vi "File read sim.vi"() -> ()   [LabVIEW 2017]
panel:
  out "Angle Array":dbl[](array[numeric])
  out "Distance Array":u32[](array[numeric])
  out "Telegram String":string
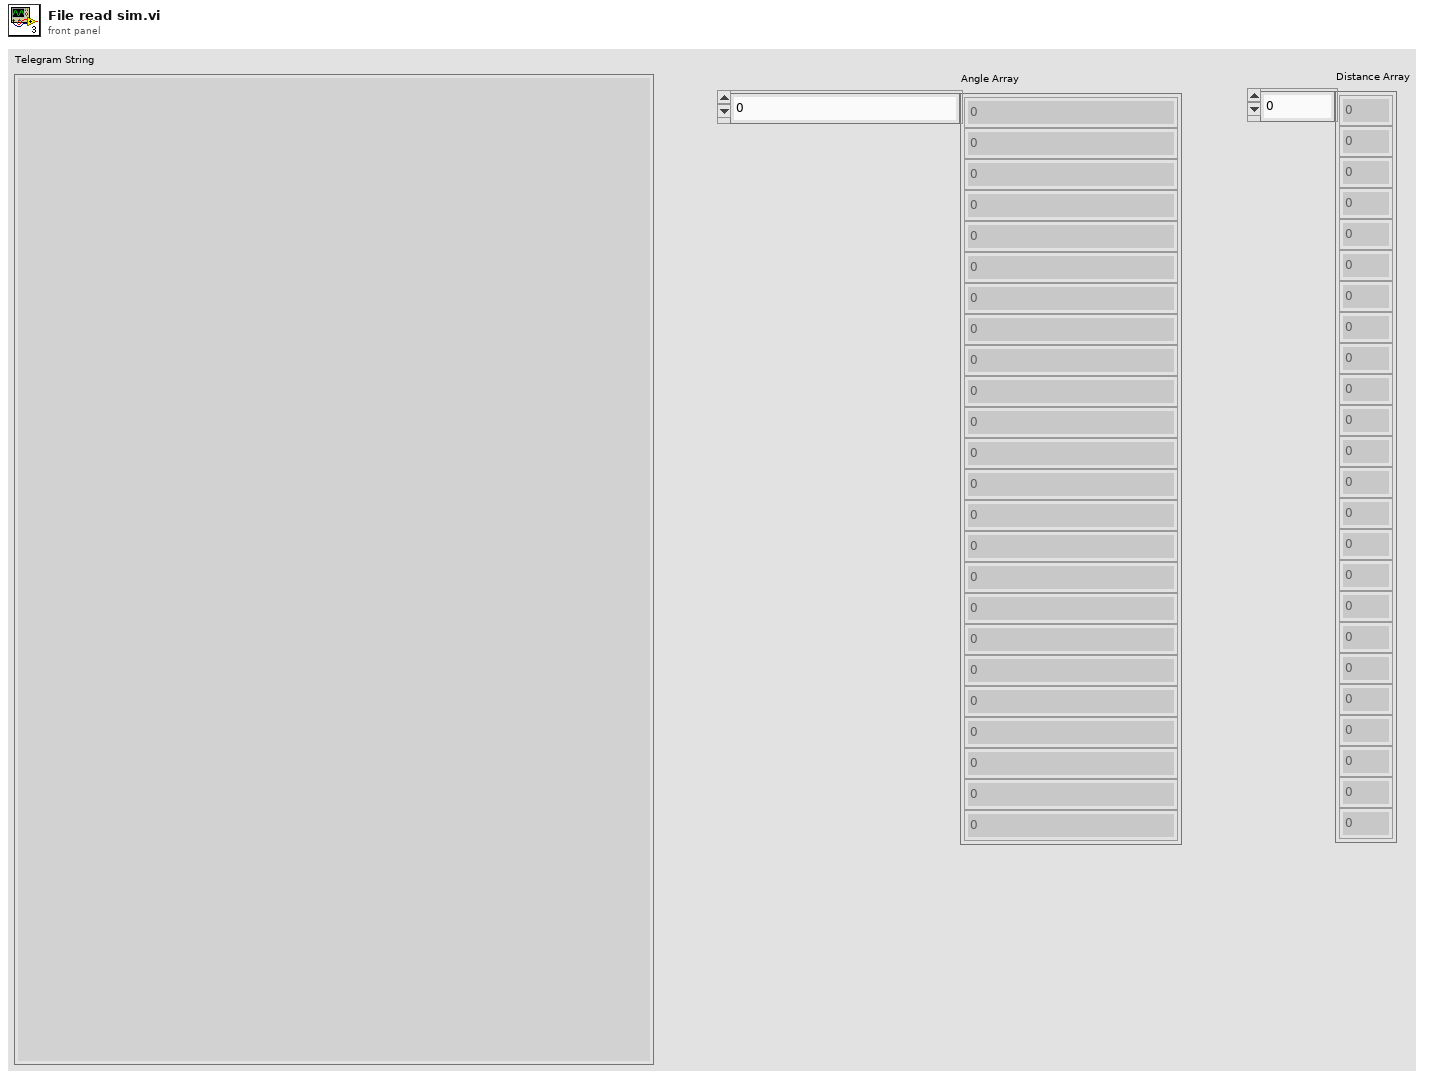
[diagram p1: front panel]
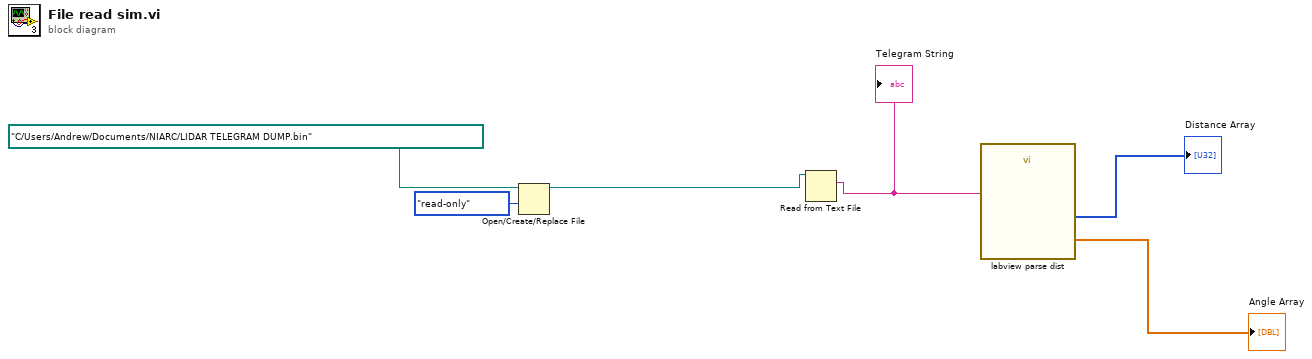
[diagram p0: block diagram]
diagram:
  n1 = Open/Create/Replace File(file path (use dialog)=path "C:/Users/Andrew/Documents/NIARC/LIDAR TELEGRAM DUMP.bin", access (0:read/write)=enum16{"read/write", "read-only", "write-only"}."read-only") -> (refnum out=w5:refnum<file>)  [unwired: 4 in, 2 out]
  n2 = Read from Text File(file (use dialog)=w5) -> (text=w6:string)  [unwired: 3 in, 3 out]
  "Telegram String" <- w6
  n3 = call "labview parse dist.vi"("Telegram String"=w6) -> ("Angle Array"=→"Angle Array":dbl[], "Distance Array"=→"Distance Array":u32[])  [unwired: 8 in]
